vi "WS1050 Delta C Calculation.vi"(8 "error in (no error)":errorcluster, 10 "DCap Target(pF)":dbl, 11 "Input":string[][](table)) -> (0 "error out":errorcluster, 1 "Total Bank Delta C(pF)":string[](array[string]), 2 "RTZ(pF)":string[][](array[string]), 3 "Delta C(pF)":string[][](array[string]), 4 "% Bank DeltaC":string[](array[string]))   [LabVIEW 2012]
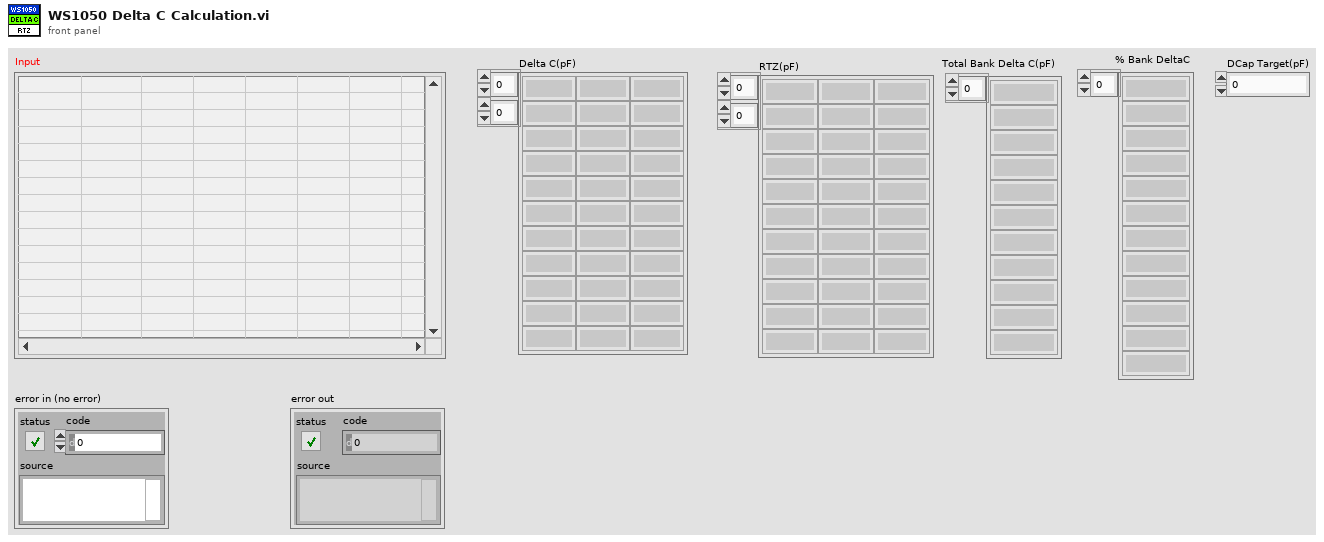
[diagram p1: front panel]
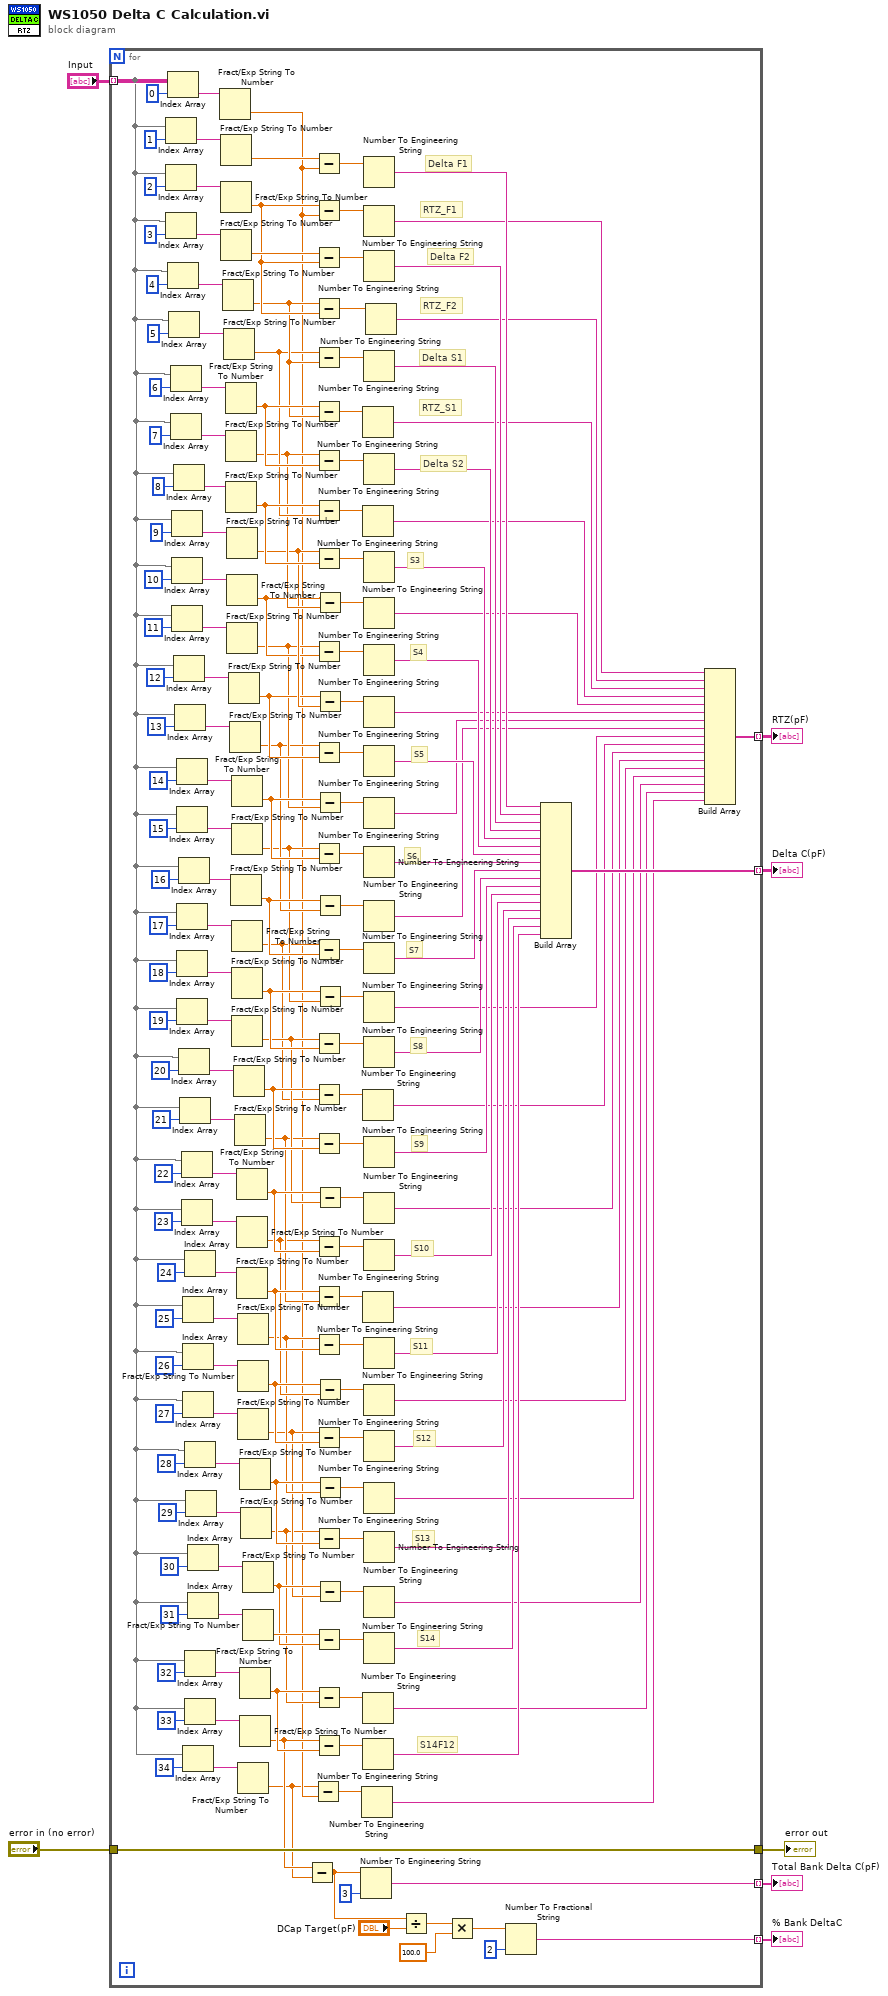
[diagram p0: block diagram]
diagram:
  n1 = for {
    tunnel: "Input" -> [w39] mode=indexing
    tunnel: [w88] -> w6 mode=indexing
    tunnel: [w21] -> w5 mode=indexing
    tunnel: "error in (no error)" -> [w20]
    tunnel: [w20] -> w3
    tunnel: [w16] -> w2 mode=indexing
    tunnel: [w8] -> w1 mode=indexing
    # "RTZ_S1"
    # "RTZ_F2"
    # "RTZ_F1"
    # "S14F12"
    # "S14"
    # "S13"
    # "S12"
    # "S11"
    # "S10"
    # "S9"
    # "S8"
    # "S7"
    # "S6"
    # "S5"
    # "S4"
    # "S3"
    # "Delta S2"
    # "Delta S1"
    # "Delta F2"
    # "Delta F1"
    n2 = Index Array(array=w39, index=1) -> (element=w188:string)
    n3 = Index Array(array=w39, index=2) -> (element=w187:string)
    n4 = Index Array(array=w39, index=3) -> (element=w184:string)
    n5 = Index Array(array=w39, index=0) -> (element=w189:string)
    n6 = Index Array(array=w39, index=4) -> (element=w183:string)
    n7 = Index Array(array=w39, index=5) -> (element=w180:string)
    n8 = Index Array(array=w39, index=6) -> (element=w179:string)
    n9 = Index Array(array=w39, index=7) -> (element=w176:string)
    n10 = Index Array(array=w39, index=9) -> (element=w163:string)
    n11 = Index Array(array=w39, index=10) -> (element=w164:string)
    n12 = Index Array(array=w39, index=11) -> (element=w167:string)
    n13 = Index Array(array=w39, index=8) -> (element=w162:string)
    n14 = Index Array(array=w39, index=12) -> (element=w168:string)
    n15 = Index Array(array=w39, index=13) -> (element=w171:string)
    n16 = Index Array(array=w39, index=14) -> (element=w172:string)
    n17 = Index Array(array=w39, index=15) -> (element=w175:string)
    n18 = Index Array(array=w39, index=17) -> (element=w107:string)
    n19 = Index Array(array=w39, index=18) -> (element=w108:string)
    n20 = Index Array(array=w39, index=19) -> (element=w111:string)
    n21 = Index Array(array=w39, index=16) -> (element=w106:string)
    n22 = Index Array(array=w39, index=20) -> (element=w112:string)
    n23 = Index Array(array=w39, index=21) -> (element=w115:string)
    n24 = Index Array(array=w39, index=22) -> (element=w116:string)
    n25 = Index Array(array=w39, index=23) -> (element=w119:string)
    n26 = Index Array(array=w39, index=25) -> (element=w132:string)
    n27 = Index Array(array=w39, index=26) -> (element=w131:string)
    n28 = Index Array(array=w39, index=27) -> (element=w128:string)
    n29 = Index Array(array=w39, index=34) -> (element=w40:string)
    n30 = Index Array(array=w39, index=24) -> (element=w133:string)
    n31 = Index Array(array=w39, index=28) -> (element=w127:string)
    n32 = Index Array(array=w39, index=32) -> (element=w99:string)
    n33 = Index Array(array=w39, index=33) -> (element=w102:string)
    n34 = Index Array(array=w39, index=29) -> (element=w124:string)
    n35 = Index Array(array=w39, index=30) -> (element=w123:string)
    n36 = Index Array(array=w39, index=31) -> (element=w120:string)
    n37 = Fract/Exp String To Number(string=w189) -> (number=w18:dbl)  [unwired: 3 in, 1 out]
    n38 = Fract/Exp String To Number(string=w188) -> (number=w191:dbl)  [unwired: 3 in, 1 out]
    n39 = Fract/Exp String To Number(string=w187) -> (number=w83:dbl)  [unwired: 3 in, 1 out]
    n40 = Fract/Exp String To Number(string=w184) -> (number=w158:dbl)  [unwired: 3 in, 1 out]
    n41 = Fract/Exp String To Number(string=w183) -> (number=w82:dbl)  [unwired: 3 in, 1 out]
    n42 = Fract/Exp String To Number(string=w180) -> (number=w79:dbl)  [unwired: 3 in, 1 out]
    n43 = Fract/Exp String To Number(string=w179) -> (number=w84:dbl)  [unwired: 3 in, 1 out]
    n44 = Fract/Exp String To Number(string=w176) -> (number=w77:dbl)  [unwired: 3 in, 1 out]
    n45 = Fract/Exp String To Number(string=w162) -> (number=w80:dbl)  [unwired: 3 in, 1 out]
    n46 = Fract/Exp String To Number(string=w163) -> (number=w75:dbl)  [unwired: 3 in, 1 out]
    n47 = Fract/Exp String To Number(string=w164) -> (number=w73:dbl)  [unwired: 3 in, 1 out]
    n48 = Fract/Exp String To Number(string=w167) -> (number=w61:dbl)  [unwired: 3 in, 1 out]
    n49 = Fract/Exp String To Number(string=w168) -> (number=w71:dbl)  [unwired: 3 in, 1 out]
    n50 = Fract/Exp String To Number(string=w171) -> (number=w60:dbl)  [unwired: 3 in, 1 out]
    n51 = Fract/Exp String To Number(string=w106) -> (number=w66:dbl)  [unwired: 3 in, 1 out]
    n52 = Fract/Exp String To Number(string=w172) -> (number=w69:dbl)  [unwired: 3 in, 1 out]
    n53 = Fract/Exp String To Number(string=w175) -> (number=w59:dbl)  [unwired: 3 in, 1 out]
    n54 = Fract/Exp String To Number(string=w107) -> (number=w58:dbl)  [unwired: 3 in, 1 out]
    n55 = Fract/Exp String To Number(string=w108) -> (number=w63:dbl)  [unwired: 3 in, 1 out]
    n56 = Fract/Exp String To Number(string=w111) -> (number=w62:dbl)  [unwired: 3 in, 1 out]
    n57 = Fract/Exp String To Number(string=w112) -> (number=w67:dbl)  [unwired: 3 in, 1 out]
    n58 = Fract/Exp String To Number(string=w115) -> (number=w55:dbl)  [unwired: 3 in, 1 out]
    n59 = Fract/Exp String To Number(string=w116) -> (number=w64:dbl)  [unwired: 3 in, 1 out]
    n60 = Fract/Exp String To Number(string=w119) -> (number=w52:dbl)  [unwired: 3 in, 1 out]
    n61 = Fract/Exp String To Number(string=w133) -> (number=w56:dbl)  [unwired: 3 in, 1 out]
    n62 = Fract/Exp String To Number(string=w132) -> (number=w49:dbl)  [unwired: 3 in, 1 out]
    n63 = Fract/Exp String To Number(string=w131) -> (number=w53:dbl)  [unwired: 3 in, 1 out]
    n64 = Fract/Exp String To Number(string=w128) -> (number=w46:dbl)  [unwired: 3 in, 1 out]
    n65 = Fract/Exp String To Number(string=w40) -> (number=w17:dbl)  [unwired: 3 in, 1 out]
    n66 = Fract/Exp String To Number(string=w127) -> (number=w50:dbl)  [unwired: 3 in, 1 out]
    n67 = Fract/Exp String To Number(string=w99) -> (number=w44:dbl)  [unwired: 3 in, 1 out]
    n68 = Fract/Exp String To Number(string=w102) -> (number=w19:dbl)  [unwired: 3 in, 1 out]
    n69 = Fract/Exp String To Number(string=w124) -> (number=w43:dbl)  [unwired: 3 in, 1 out]
    n70 = Fract/Exp String To Number(string=w123) -> (number=w47:dbl)  [unwired: 3 in, 1 out]
    n71 = Fract/Exp String To Number(string=w120) -> (number=w143:dbl)  [unwired: 3 in, 1 out]
    n72 = Subtract(x=w19, y=w17) -> (x-y=w14:dbl)
    n73 = Subtract(x=w17, y=w18) -> (x-y=w42:dbl)
    n74 = Subtract(x=w191, y=w18) -> (x-y=w190:dbl)
    n75 = Subtract(x=w83, y=w18) -> (x-y=w87:dbl)
    n76 = Subtract(x=w158, y=w83) -> (x-y=w159:dbl)
    n77 = Subtract(x=w82, y=w83) -> (x-y=w86:dbl)
    n78 = Subtract(x=w79, y=w82) -> (x-y=w157:dbl)
    n79 = Subtract(x=w84, y=w82) -> (x-y=w85:dbl)
    n80 = Subtract(x=w77, y=w84) -> (x-y=w156:dbl)
    n81 = Subtract(x=w80, y=w79) -> (x-y=w81:dbl)
    n82 = Subtract(x=w75, y=w80) -> (x-y=w155:dbl)
    n83 = Subtract(x=w61, y=w73) -> (x-y=w154:dbl)
    n84 = Subtract(x=w60, y=w71) -> (x-y=w153:dbl)
    n85 = Subtract(x=w59, y=w69) -> (x-y=w152:dbl)
    n86 = Subtract(x=w58, y=w66) -> (x-y=w105:dbl)
    n87 = Subtract(x=w62, y=w63) -> (x-y=w136:dbl)
    n88 = Subtract(x=w67, y=w58) -> (x-y=w68:dbl)
    n89 = Subtract(x=w55, y=w67) -> (x-y=w137:dbl)
    n90 = Subtract(x=w52, y=w64) -> (x-y=w138:dbl)
    n91 = Subtract(x=w56, y=w55) -> (x-y=w57:dbl)
    n92 = Subtract(x=w49, y=w56) -> (x-y=w139:dbl)
    n93 = Subtract(x=w46, y=w53) -> (x-y=w140:dbl)
    n94 = Subtract(x=w43, y=w50) -> (x-y=w141:dbl)
    n95 = Subtract(x=w143, y=w47) -> (x-y=w142:dbl)
    n96 = Subtract(x=w44, y=w43) -> (x-y=w45:dbl)
    n97 = Subtract(x=w19, y=w44) -> (x-y=w98:dbl)
    n98 = Subtract(x=w73, y=w77) -> (x-y=w78:dbl)
    n99 = Subtract(x=w71, y=w75) -> (x-y=w76:dbl)
    n100 = Subtract(x=w69, y=w61) -> (x-y=w74:dbl)
    n101 = Subtract(x=w66, y=w60) -> (x-y=w72:dbl)
    n102 = Subtract(x=w63, y=w59) -> (x-y=w70:dbl)
    n103 = Subtract(x=w64, y=w62) -> (x-y=w65:dbl)
    n104 = Subtract(x=w53, y=w52) -> (x-y=w54:dbl)
    n105 = Subtract(x=w50, y=w49) -> (x-y=w51:dbl)
    n106 = Subtract(x=w47, y=w46) -> (x-y=w48:dbl)
    n107 = Number To Engineering String(2:i16 3 ("precision (6)"), 4:w14) -> (0:w16:string)  [unwired: 2 in]
    n108 = Number To Engineering String(4:w42) -> (0:w22:string)  [unwired: 3 in]
    n109 = Number To Engineering String(4:w85) -> (0:w36:string)  [unwired: 3 in]
    n110 = Number To Engineering String(4:w81) -> (0:w35:string)  [unwired: 3 in]
    n111 = Number To Engineering String(4:w68) -> (0:w29:string)  [unwired: 3 in]
    n112 = Number To Engineering String(4:w57) -> (0:w27:string)  [unwired: 3 in]
    n113 = Number To Engineering String(4:w45) -> (0:w23:string)  [unwired: 3 in]
    n114 = Number To Engineering String(4:w98) -> (0:w89:string)  [unwired: 3 in]
    n115 = Number To Engineering String(4:w190) -> (0:w151:string)  [unwired: 3 in]
    n116 = Number To Engineering String(4:w87) -> (0:w38:string)  [unwired: 3 in]
    n117 = Number To Engineering String(4:w159) -> (0:w150:string)  [unwired: 3 in]
    n118 = Number To Engineering String(4:w157) -> (0:w149:string)  [unwired: 3 in]
    n119 = Number To Engineering String(4:w156) -> (0:w148:string)  [unwired: 3 in]
    n120 = Number To Engineering String(4:w155) -> (0:w147:string)  [unwired: 3 in]
    n121 = Number To Engineering String(4:w78) -> (0:w34:string)  [unwired: 3 in]
    n122 = Number To Engineering String(4:w154) -> (0:w146:string)  [unwired: 3 in]
    n123 = Number To Engineering String(4:w76) -> (0:w33:string)  [unwired: 3 in]
    n124 = Number To Engineering String(4:w153) -> (0:w145:string)  [unwired: 3 in]
    n125 = Number To Engineering String(4:w74) -> (0:w32:string)  [unwired: 3 in]
    n126 = Number To Engineering String(4:w152) -> (0:w144:string)  [unwired: 3 in]
    n127 = Number To Engineering String(4:w72) -> (0:w31:string)  [unwired: 3 in]
    n128 = Number To Engineering String(4:w105) -> (0:w97:string)  [unwired: 3 in]
    n129 = Number To Engineering String(4:w70) -> (0:w30:string)  [unwired: 3 in]
    n130 = Number To Engineering String(4:w136) -> (0:w96:string)  [unwired: 3 in]
    n131 = Number To Engineering String(4:w137) -> (0:w95:string)  [unwired: 3 in]
    n132 = Number To Engineering String(4:w65) -> (0:w28:string)  [unwired: 3 in]
    n133 = Number To Engineering String(4:w138) -> (0:w94:string)  [unwired: 3 in]
    n134 = Number To Engineering String(4:w139) -> (0:w93:string)  [unwired: 3 in]
    n135 = Number To Engineering String(4:w54) -> (0:w26:string)  [unwired: 3 in]
    n136 = Number To Engineering String(4:w140) -> (0:w92:string)  [unwired: 3 in]
    n137 = Number To Engineering String(4:w51) -> (0:w25:string)  [unwired: 3 in]
    n138 = Number To Engineering String(4:w141) -> (0:w91:string)  [unwired: 3 in]
    n139 = Number To Engineering String(4:w48) -> (0:w24:string)  [unwired: 3 in]
    n140 = Number To Engineering String(4:w142) -> (0:w90:string)  [unwired: 3 in]
    n141 = Number To Engineering String(4:w86) -> (0:w37:string)  [unwired: 3 in]
    n142 = Divide(x=w14, y="DCap Target(pF)") -> (x/y=w12:dbl)
    n143 = Multiply(x=w12, y=100.0) -> (x*y=w10:dbl)
    n144 = Number To Fractional String(number=w10, precision (6)=i16 2) -> (F-format string=w8:string)  [unwired: 2 in]
    n145 = Build Array(w151, w150, w149, w148, w147, w146, w145, w144, w97, w96, w95, w94, w93, w92, w91, w90, w89) -> (w88:string[])
    n146 = Build Array(w38, w37, w36, w35, w34, w33, w32, w31, w30, w29, w28, w27, w26, w25, w24, w23, w22) -> (w21:string[])
  }
  "Delta C(pF)" <- w6
  "RTZ(pF)" <- w5
  "error out" <- w3
  "Total Bank Delta C(pF)" <- w2
  "% Bank DeltaC" <- w1
